vi "Initialize.vi"(8 "error in (no error)":errorcluster, 11 "Laser_Oxxius in":refnum<class "Laser_Oxxius.lvclass">) -> (0 "error out":errorcluster, 3 "Laser_Oxxius out":refnum<class "Laser_Oxxius.lvclass">)   [LabVIEW 2020, in "Laser_Oxxius.lvlib" / "Laser_Oxxius.lvclass"]
uses:
  Laser_Oxxius.lvclass
  D:/Daguan/Development/MMicroscopyAF/Model/Hardware Layer/Real Hardware/Laser_Oxxius/Laser_Oxxius/Dependency/Oxxius_Boxx.dll
  Dependency/Oxxius_Boxx.dll
  Laser_Oxxius.lvclass/Laser_Oxxius.ctl
  Hardware Abstraction Layer/Component/Laser/Laser/Laser.lvclass
panel:
  in  "785 Power":dbl caption="LAS-03914" min=0.0 max=200.0
  in  "647 Power":sgl caption="LAS-05914"
  in  "561 Power":dbl caption="LAS-05858" min=0.0 max=200.0
  in  "532 Power":sgl caption="LAS-05886" min=0 max=200
  in  "488 Power":dbl caption="LAS-06030" min=0.0 max=200.0
  in  "405 Power":dbl caption="LAS-05997" min=0.0 max=200.0
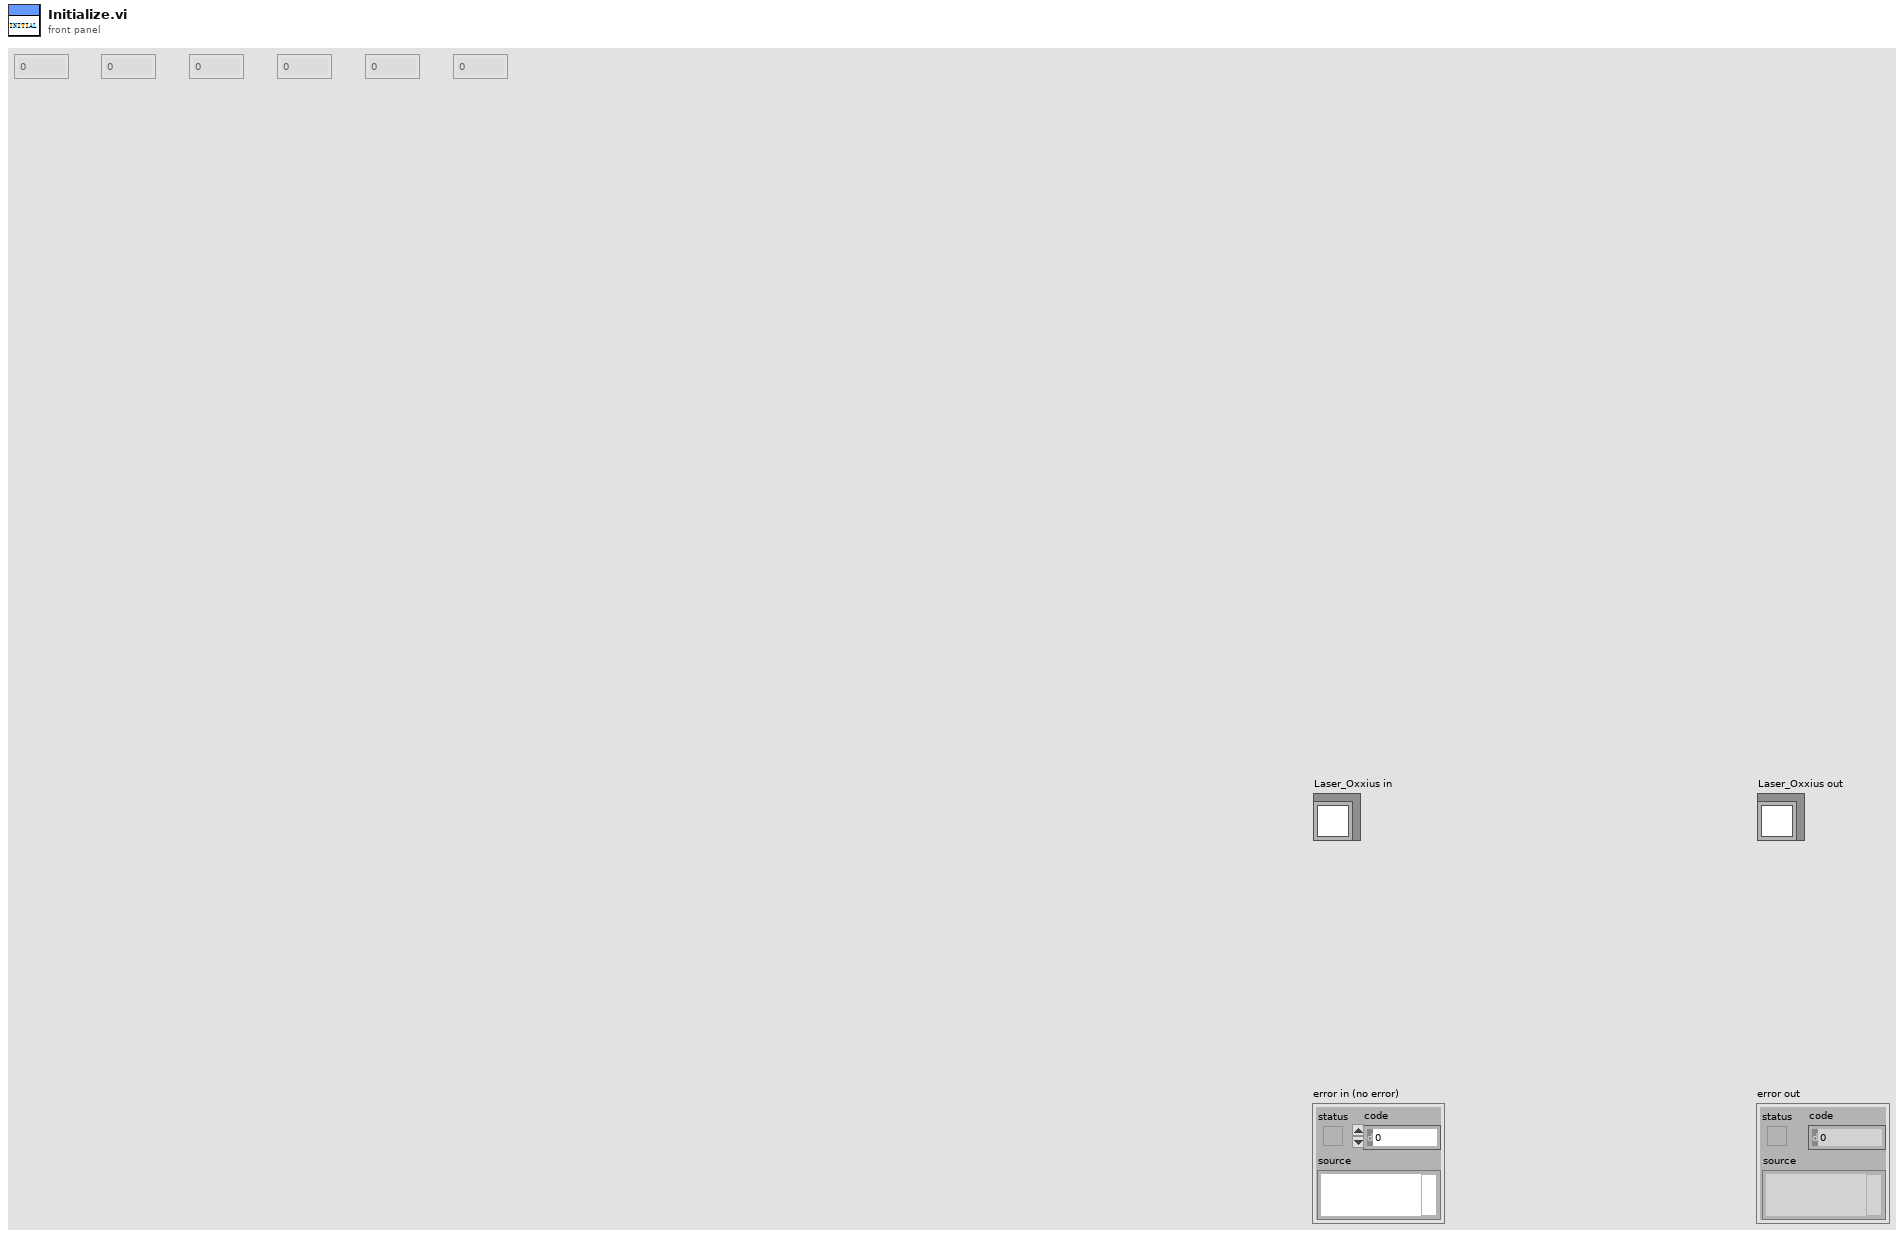
[diagram p1: front panel]
types:
  T1 = typedef "DataListener.lvclass/DataExchange.ctl" = cluster{"Source":string, "Destination":string, "Description":string, "value":variant}
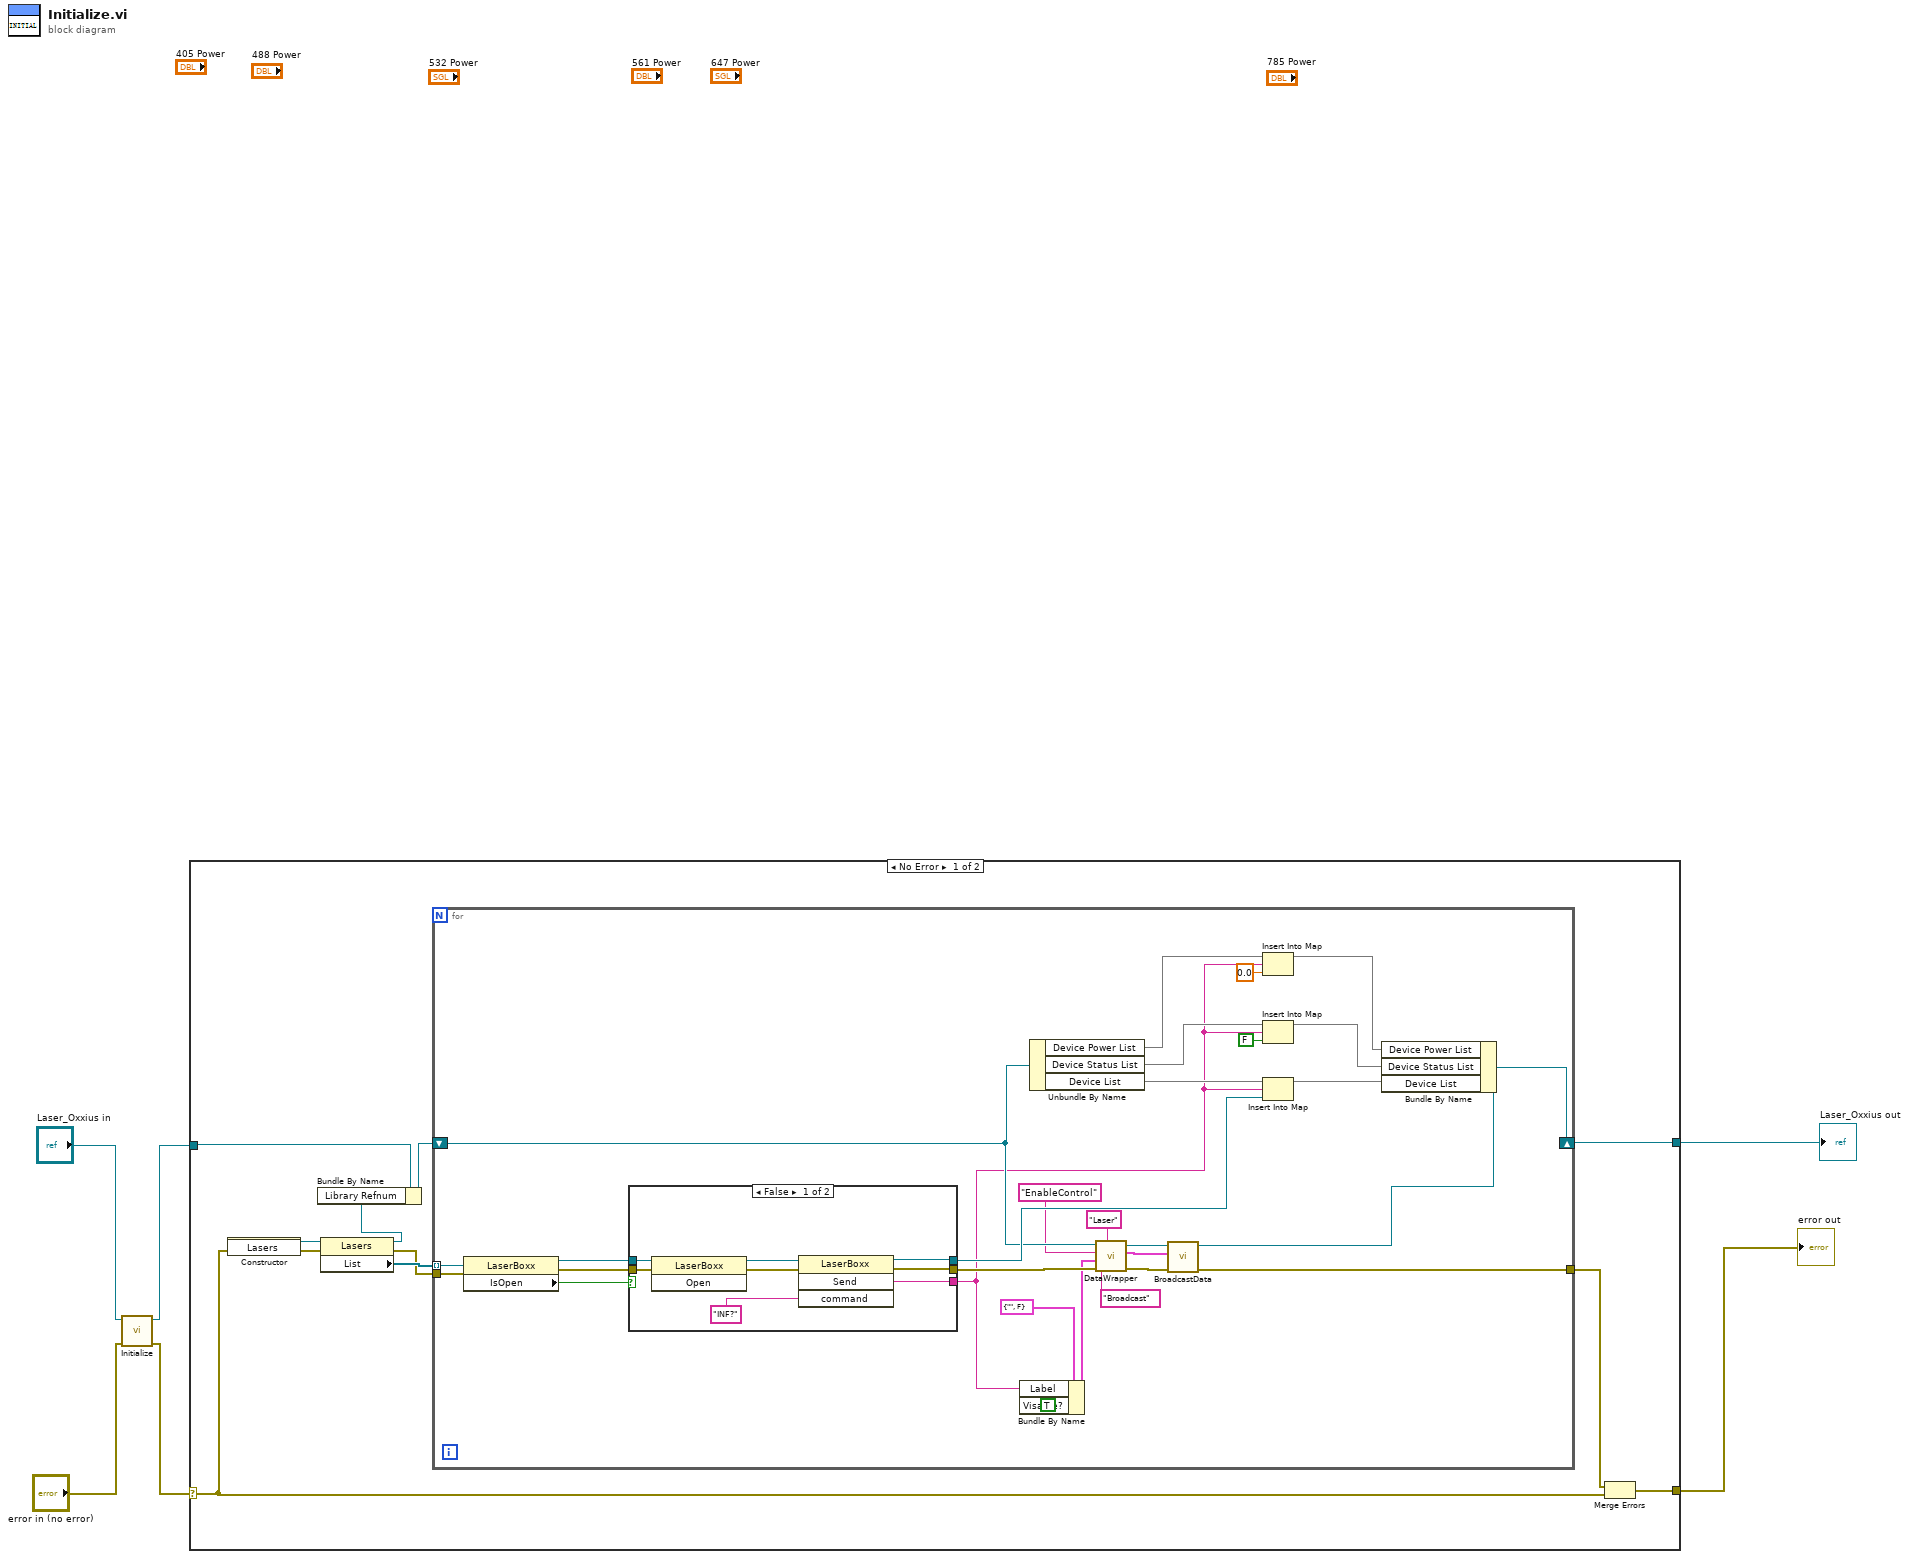
[diagram p0: block diagram]
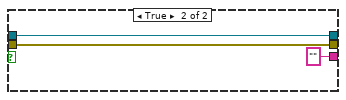
[diagram p2: hidden frame]
diagram:
  n1 = call-parent "Initialize.vi"("error in (no error)"="error in (no error)", "Laser in"="Laser_Oxxius in") -> ("error out"=w2:errorcluster, "Laser out"=w1:refnum<class "Laser_Oxxius.lvclass">)  [unwired: 8 in]
  n2 = case shown="No Error" w2 {
    selector: w2 -> [w10 w59]
    tunnel: [w17 w59] -> w5
    tunnel: [w11 w58] -> w6
    tunnel: w1 -> [w9 w58]
    frame No Error {
      n3 = constructor class="Lasers"(error in=w10) -> (reference out=w15:refnum<k24>, error out=w14:errorcluster)  [unwired: 2 in, 1 out]
      n4 = property class="Lasers"(reference=w15, error in=w14) -> (reference out=w7:refnum<k24>, error out=w13:errorcluster, "List"=w16:refnum<k24>[])
      n5 = Bundle By Name(cluster=w9, "Library Refnum"=w7) -> (w8:refnum<class "Laser_Oxxius.lvclass">)
      n6 = for {
        tunnel: w16 -> [w46] mode=indexing
        tunnel: w13 -> [w45]
        tunnel: [w35] -> w12
        shift-right: [w41] -> w11
        shift-left: w8 -> [w32]
        n7 = property class="LaserBoxx"(reference=w46, error in=w45) -> (reference out=w44:refnum<k24>, error out=w43:errorcluster, "IsOpen"=w42:bool)
        n8 = case shown="False" w42 {
          tunnel: w43 -> [w54 w57]
          tunnel: w44 -> [w53 w56]
          tunnel: [w48 w57] -> w37
          tunnel: [w49 w56] -> w39
          tunnel: [w47 "" ("Send")] -> w18
          frame False {
            n9 = invoke class="LaserBoxx" method="Open"(reference=w53, error in=w54) -> (reference out=w50:refnum<k24>, error out=w51:errorcluster)  [unwired: 1 in, 1 out]
            n10 = invoke class="LaserBoxx" method="Send"(reference=w50, error in=w51, "command"="INF?") -> (reference out=w49:refnum<k24>, error out=w48:errorcluster, "Send"=w47:string)  [unwired: 1 in, 1 out]
          }
          frame True {
          }
        }
        n11 = Bundle By Name(cluster=cluster{"Label":string, "Visable?":bool} {"Label"="", "Visable?"=FALSE} ("event data"), "Label"=w18, "Visable?"=TRUE) -> (w26:cluster{"Label":string, "Visable?":bool})
        n12 = Unbundle By Name(w32) -> ("Device Power List"=w24:map{string, dbl}, "Device Status List"=w22:map{string, bool}, "Device List"=w40:map{string, refnum<k24>})
        n13 = call-dynamic "DataWrapper.vi"("Destination"="Broadcast" ("Type"), "Source"="Laser", "error in (no error)"=w37, "value"=w26, "Description"="EnableControl" ("Target"), "GRMActor in"=w32) -> ("error out"=w36:errorcluster, "DataExchange"=w31:T1, "GRMActor out"=w34:refnum<class "Laser_Oxxius.lvclass">)  [unwired: 3 in]
        n14 = call-dynamic "BroadcastData.vi"("error in (no error)"=w36, "DataExchange"=w31, "GRMActor in"=w34) -> ("error out"=w35:errorcluster, "GRMActor out"=w33:refnum<class "Laser_Oxxius.lvclass">)  [unwired: 7 in]
        n15 = Insert Into Map(map in=w24, key=w18, value=0.0) -> (map out=w23:map{string, dbl})  [unwired: 2 out]
        n16 = Insert Into Map(map in=w22, key=w18, value=FALSE) -> (map out=w21:map{string, bool})  [unwired: 2 out]
        n17 = Insert Into Map(map in=w40, key=w18, value=w39) -> (map out=w38:map{string, refnum<k24>})  [unwired: 2 out]
        n18 = Bundle By Name(cluster=w33, "Device Power List"=w23, "Device Status List"=w21, "Device List"=w38) -> (w41:refnum<class "Laser_Oxxius.lvclass">)
      }
      n19 = Merge Errors(w12, w10) -> (w17:errorcluster)
    }
    frame Error {
    }
  }
  "error out" <- w5
  "Laser_Oxxius out" <- w6
